vi "Read Settings.vi"(8 "error in (no error)":errorcluster, 11 "INL PID in":refnum<class "INL PID.lvclass">) -> (0 "error out":errorcluster, 2 "INL PID":T1={"Sampling Frequency"=0.5, "Integration Time"=50.0, "Integration Periods"=50, "Grid Voltage"=50.0}, 3 "INL PID out":refnum<class "INL PID.lvclass">)   [LabVIEW 2011, in "INL PID.lvclass"]
uses:
  INL PID.lvclass
  Settings.ctl
  INL PID.lvclass/INL PID.ctl
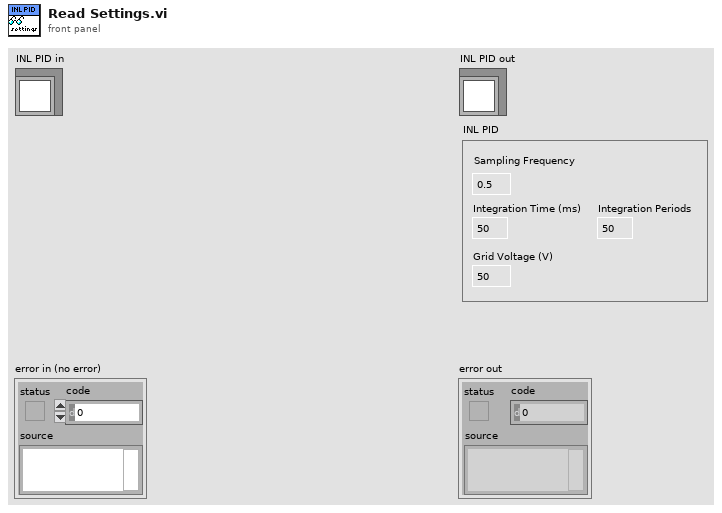
[diagram p1: front panel]
types:
  T1 = typedef "INL PID.lvclass/Settings.ctl" = cluster{"Sampling Frequency":dbl, "Integration Time":dbl, "Integration Periods":u8, "Grid Voltage":dbl}
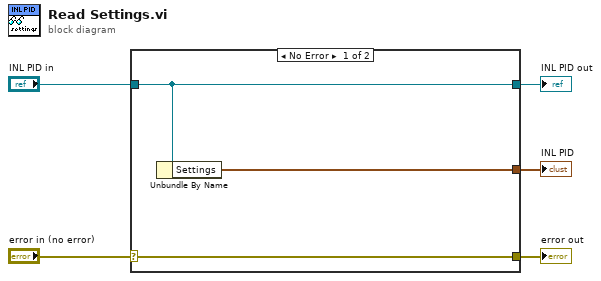
[diagram p0: block diagram]
diagram:
  n1 = case shown="No Error" "error in (no error)" {
    selector: "error in (no error)" -> [w8 w9]
    tunnel: [w8 w9] -> w4
    tunnel: [w7 w10] -> w2
    tunnel: "INL PID in" -> [w7 w10]
    tunnel: [w6 _] -> w1
    frame No Error {
      n2 = Unbundle By Name(w7) -> ("Settings"=w6:T1)
    }
    frame Error {
    }
  }
  "error out" <- w4
  "INL PID out" <- w2
  "INL PID" <- w1
